vi "Reset Quadrature.vi"(8 "error in":errorcluster, 10 "Forward Position":i32, 11 "Enum":T1) -> (0 "error out":errorcluster, 3 "Encoder Offset":i32)   [LabVIEW 2016]
uses:
  Control Files/SwerveMotors.ctl
  Main/Robot Global Data.vi
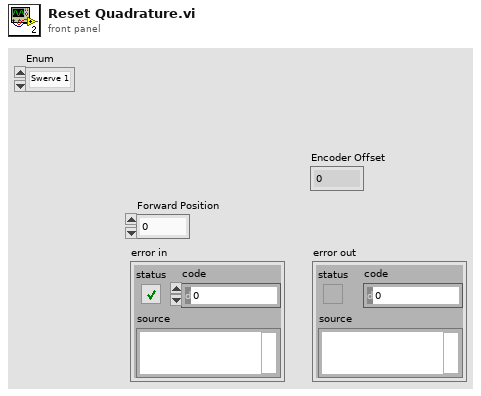
[diagram p1: front panel]
types:
  T1 = typedef "SwerveMotors.ctl" = enum16{"Swerve 1", "Swerve 2", "Swerve 3", "Swerve 4"}
  T2 = typedef "WPI_MotorControlDeviceRef.ctl" = cluster{"DeviceStatus":errorcluster, "Type":T3, "PWM":cluster{"PWM Channel":T4, "DeadBand":T5}, "CAN":cluster{"Device Number":u8, "SetOutput VI Ref":variant, "GetOutput VI Ref":variant, "Enable VI Ref":variant, "Disable VI Ref":variant, "Data":variant}, "Invert":bool}
  T3 = typedef "WPI_MotorControlType.ctl" = enum16{"PWM", "CAN"}
  T4 = typedef "FPGA_DIOPWMChannel.ctl" = enum8{"PWM 0", "PWM 1", "PWM 2", "PWM 3", "PWM 4", "PWM 5", "PWM 6", "PWM 7", "PWM 8", "PWM 9", "PWM MXP 0", "PWM MXP 1", "PWM MXP 2", "PWM MXP 3", "PWM MXP 4", "PWM MXP 5", "PWM MXP 6", "PWM MXP 7", "PWM MXP 8", "PWM MXP 9", "Invalid"}
  T5 = typedef "WPI_PWMDeadband.ctl" = cluster{"Name":string, "maxPositivePwm":i32, "minPositivePwm":i32, "centerPwm":i32, "maxNegativePwm":i32, "minNegativePwm":i32, "angularRange":u16}
  T6 = typedef "WPI_CANTalonSRX_GlobalStatus.ctl" = cluster{"Applied Throttle":dbl, "Module Enabled":bool, "CAN Error":errorcluster, "Closed Loop Error":dbl, "Forward Limit Switch Closed":bool, "Reverse Limit Switch Closed":bool, "Sensor Position":dbl, "Sensor Velocity":dbl, "Current":dbl, "Sticky Fault - Over Temp":bool, "Sticky Fault - Under Voltage":bool, "Sticky Fault - Forward Limit":bool, "Sticky Fault - Reverse Limit":bool, "Sticky Fault - Forward Soft Limit":bool, "Sticky Fault - Reverse Soft Limit":bool, "Brake is Enabled":bool, "Encoder Position":dbl, "Encoder Velocity":dbl, "Encoder Index Count":dbl, "Encoder A Pin State":bool, "Encoder B Pin State":bool, "Encoder Index Pin State":bool, "Analog In":dbl, "Analog In Velocity":dbl, "Temperature (C)":dbl, "Battery Voltage":dbl, "Control 5 Is Supported":bool, "Current Profile Slot Select":dbl, "Pos Div 8":bool, "Vel Div 4":bool, "Pulse Width Position":i32, "Pulse Width Velocity":i32, "Pulse Width Rise To Rise (us)":i32, "Pulse Width Rise To Fall (us)":i32, "Mot Prof Active Is Under Run":bool, "Mot Prof Active Has Under Run":bool, "Mot Prof Active Is Last":bool, "Mot Prof Active Velocity Only":bool, "Mot Prof Active Is Valid":bool, "Mot Prof Buffer Is Full":bool, "Mot Prof Active Profile Slot Select":i32, "Mot Prof NextID":i32, "Mot Prof Count":i32, "Mot Prof Active Velocity":dbl, "Mot Prof Active Position":dbl, "Mot Prof Output Enable":i32}
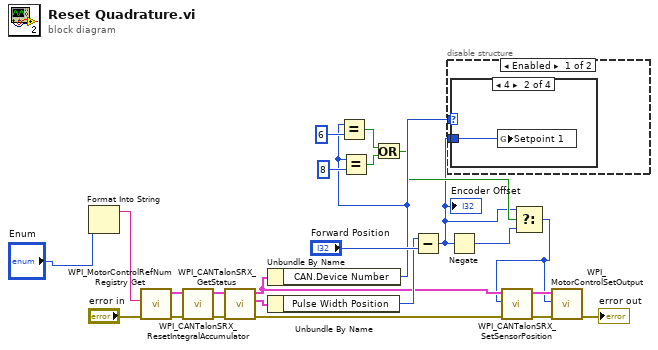
[diagram p0: block diagram]
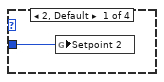
[diagram p2: hidden frame]
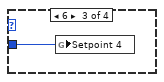
[diagram p3: hidden frame]
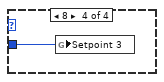
[diagram p4: hidden frame]
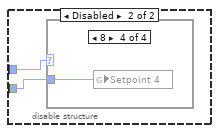
[diagram p5: hidden frame]
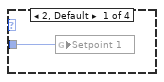
[diagram p6: hidden frame]
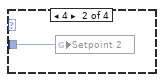
[diagram p7: hidden frame]
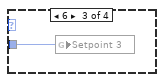
[diagram p8: hidden frame]
diagram:
  n1 = Format Into String("Enum") -> (resulting string=w2:string)  [unwired: 3 in, 1 out]
  n2 = call <vilib>:"WPI_MotorControlRefNum Registry Get.vi"("error in (no error)"="error in", "refnum name"=w2) -> ("error out"=w18:errorcluster, "MotorControlDevRef"=w19:T2)  [unwired: 8 in]
  n3 = call <vilib>:"WPI_CANTalonSRX_ResetIntegralAccumulator.vi"("error in (no error)"=w18, "CAN Talon SRX Ref"=w19) -> ("error out"=w16:errorcluster, "CAN Talon SRX Ref"=w17:T2)  [unwired: 8 in]
  n4 = call <vilib>:"WPI_CANTalonSRX_GetStatus.vi"("error in (no error)"=w16, "CAN Talon SRX Ref"=w17) -> ("error out"=w20:errorcluster, "Talon SRX Status"=w23:T6, "CAN Talon SRX Ref"=w13:T2)  [unwired: 7 in]
  n5 = Unbundle By Name(w13) -> ("CAN.Device Number"=w7:u8)
  n6 = Unbundle By Name(w23) -> ("Pulse Width Position"=w21:i32)
  n7 = Equal?(x=w7, y=u8 6) -> (x = y?=w9:bool)
  n8 = Equal?(x=w7, y=u8 8) -> (x = y?=w8:bool)
  n9 = Or(x=w9, y=w8) -> (x .or. y?=w6:bool)
  n10 = Subtract(x=w21, y="Forward Position") -> (x-y=w5:i32)
  "Encoder Offset" <- w5
  n11 = disable-structure shown="Enabled" {
    disable-tunnel: w7 -> [w26 w32]
    disable-tunnel: w5 -> [w25 w31]
    frame Enabled {
      n12 = case shown="4" w26 {
        tunnel: w25 -> [w27 w28 w29 w30]
        frame 2, Default {
          n13 = global write "Robot Global Data.vi" "Setpoint 2"(w27) -> ()
        }
        frame 4 {
          n14 = global write "Robot Global Data.vi" "Setpoint 1"(w28) -> ()
        }
        frame 6 {
          n15 = global write "Robot Global Data.vi" "Setpoint 4"(w29) -> ()
        }
        frame 8 {
          n16 = global write "Robot Global Data.vi" "Setpoint 3"(w30) -> ()
        }
      }
    }
    frame Disabled {
      n17 = case shown="8" w32 {
        tunnel: w31 -> [w33 w34 w35 w36]
        frame 2, Default {
          n18 = global write "Robot Global Data.vi" "Setpoint 1"(w33) -> ()
        }
        frame 4 {
          n19 = global write "Robot Global Data.vi" "Setpoint 2"(w34) -> ()
        }
        frame 6 {
          n20 = global write "Robot Global Data.vi" "Setpoint 3"(w35) -> ()
        }
        frame 8 {
          n21 = global write "Robot Global Data.vi" "Setpoint 4"(w36) -> ()
        }
      }
    }
  }
  n22 = Negate(x=w5) -> (-x=w4:i32)
  n23 = Select(t=w5, s=w6, f=w4) -> (s? t:f=w3:i32)
  n24 = call <vilib>:"WPI_CANTalonSRX_SetSensorPosition.vi"("error in (no error)"=w20, "New Sensor Position"=w3, "CAN Talon SRX Ref"=w13) -> ("error out"=w14:errorcluster, "CAN Talon SRX Ref"=w15:T2)  [unwired: 7 in]
  n25 = call <vilib>:"WPI_MotorControlSetOutput.vi"("error in (no error)"=w14, "Output"=w3, "MotorControlDevRef"=w15) -> ("error out"=→"error out":errorcluster)  [unwired: 6 in, 2 out]
